vi "Program23.vi"() -> ()   [LabVIEW 2020]
panel:
  out "Wynikowa 3":string[](array[string])
  out "Wynikowa 1":string[](array[string])
  out "Wynikowa 2":string[](array[string])
  out "Spleciona":string[](array[string])
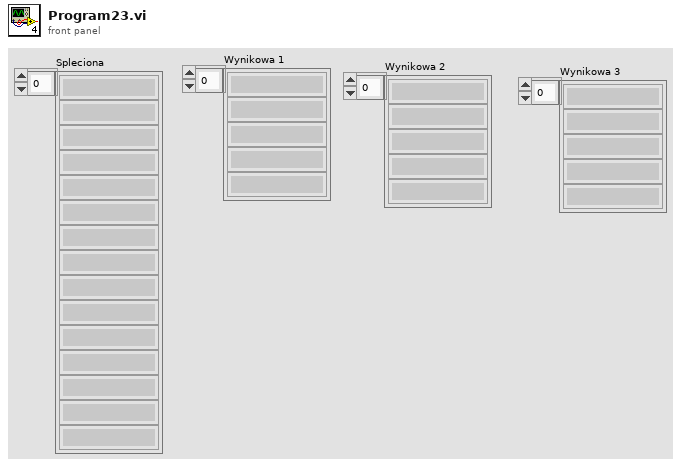
[diagram p1: front panel]
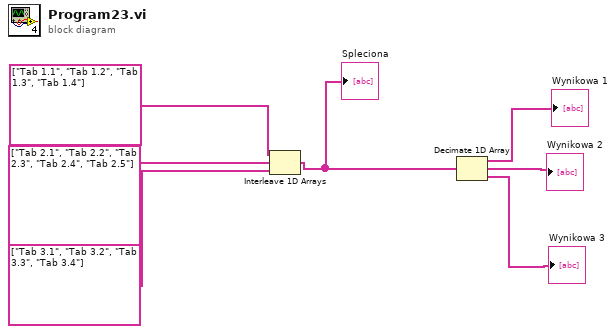
[diagram p0: block diagram]
diagram:
  n1 = Interleave 1D Arrays(string[] ["Tab 1.1", "Tab 1.2", "Tab 1.3", "Tab 1.4"], string[] ["Tab 2.1", "Tab 2.2", "Tab 2.3", "Tab 2.4", "Tab 2.5"], string[] ["Tab 3.1", "Tab 3.2", "Tab 3.3", "Tab 3.4"]) -> (w4:string[])
  "Spleciona" <- w4
  n2 = Decimate 1D Array(w4) -> (→"Wynikowa 1":string[], →"Wynikowa 2":string[], →"Wynikowa 3":string[])
